vi "Write settings.vi"(7 "force saving?":bool, 8 "error in (no error)":errorcluster, 11 "ImagingModeSPIM in":refnum<class "InVivo_ImagingModeSPIM.lvclass">) -> (0 "error out":errorcluster, 1 "cancelled":bool, 2 "settings name":string, 3 "ImagingModeSPIM out":refnum<class "InVivo_ImagingModeSPIM.lvclass">)   [LabVIEW 2012, in "InVivo_ImagingModeSPIM.lvclass"]
uses:
  InVivo_ImagingModeSPIM.lvclass
  <vilib>/Distrio/Murmex/Murmex/Murmex.lvclass
  InVivo_ImagingModeSPIM.lvclass/InVivo_ImagingModeSPIM.ctl
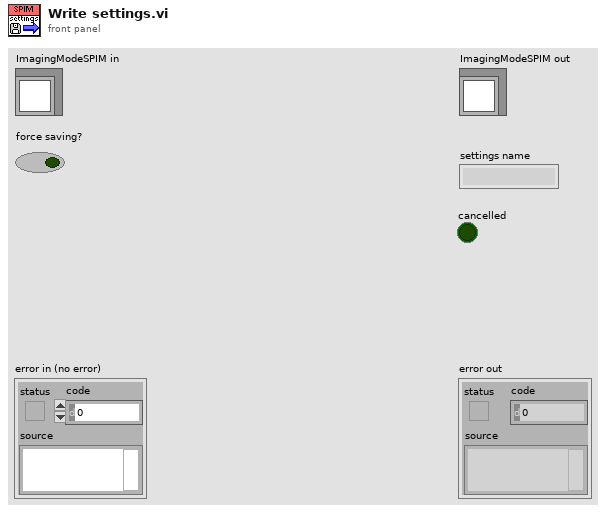
[diagram p1: front panel]
types:
  T1 = typedef "InVivo_ImagingModeSPIM.lvclass/settings_cluster.ctl" = cluster{"Frequency":dbl[unit], "Amplitude1":dbl[unit], "Phase1":dbl[unit], "DC offset1":dbl[unit], "Amplitude2":dbl[unit], "Phase2":dbl[unit], "DC offset2":dbl[unit], "Waveform type":T2, "HSYNC pulses":dbl, "pulses per pixel":i32, "digital ratio":dbl, "DC offset3":dbl[unit], "Amplitude3":dbl[unit], "Phase3":dbl[unit], "AOTFamplitude":dbl[unit], "AOTFoffset":dbl[unit], "AOTFphase":dbl[unit], "AOTFwaveform":T3, "Startaotf":bool}
  T2 = typedef "InVivo_ImagingModeSPIM.lvclass/waveform_enum.ctl" = enum16{"triangular", "sawtooth", "sinusodial"}
  T3 = typedef "InVivo_ImagingModeSPIM.lvclass/Control 4.ctl" = enum16{"Triangular", "Sawtooth", "Sinusoidal"}
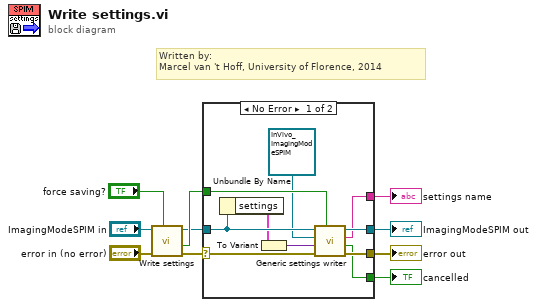
[diagram p0: block diagram]
diagram:
  # "Written by:\nMarcel van 't Hoff, University of Florence, 2014"
  n1 = call-parent "Write settings.vi"("force saving?"="force saving?", "error in (no error)"="error in (no error)", "Murmex in"="ImagingModeSPIM in") -> ("error out"=w7:errorcluster, "cancelled"=w6:bool, "Murmex out"=w5:refnum<class "InVivo_ImagingModeSPIM.lvclass">)  [unwired: 5 in, 1 out]
  n2 = case shown="No Error" w7 {
    selector: w7 -> [w20 w22]
    tunnel: [w19 w22] -> w1
    tunnel: [w17 w21] -> w3
    tunnel: w5 -> [w18 w21]
    tunnel: [w16 _] -> w4
    tunnel: [w15 _] -> w2
    tunnel: w6 -> [w14 _]
    frame No Error {
      n3 = Unbundle By Name(w18) -> ("settings"=w13:T1)
      n4 = To Variant(anything=w13) -> (Variant=w12:variant)
      n5 = call <vilib>:"Generic settings writer.vi"("force saving?"=w14, "error in (no error)"=w20, "settings"=w12, "inheritance level"=refnum<class "InVivo_ImagingModeSPIM.lvclass"> refnum ("ImagingModeSPIM"), "Murmex in"=w18) -> ("error out"=w19:errorcluster, "cancelled"=w15:bool, "settings name"=w16:string, "Murmex out"=w17:refnum<class "InVivo_ImagingModeSPIM.lvclass">)  [unwired: 3 in]
    }
    frame Error {
    }
  }
  "error out" <- w1
  "ImagingModeSPIM out" <- w3
  "settings name" <- w4
  "cancelled" <- w2
